vi "XVA-DSE1-dist.vi"(8 "err in":errorcluster, 10 "X-VA (e)":T2, 11 "p_LN":T1) -> (0 "err out":errorcluster, 2 "X-VA (s)":T2, 3 "p_LN (s)":T1)   [LabVIEW 2010, in "lv_04.lvlib"]
uses:
  lv_04.lvlib
  lv_02/p_5E1_LN.ctl
  commandes/cX.ctl
  commandes/cSTA_varid.ctl
  commandes/c_TDMS_ch_variable.ctl
  commandes/c_TDMS_ch_donnees.ctl
  commandes/c0-var-n.ctl
  commandes/cSTA_num_do_cr.ctl
  commandes/c02-do-num.ctl
  commandes/c04-stat-num.ctl
  commandes/cSTA_txt_do_cr.ctl
  commandes/c02-do-txt.ctl
  commandes/c04-stat-txt.ctl
  commandes/cSTA_dist.ctl
  commandes/c03-dist-S.ctl
  commandes/c0-dist-xy.ctl
  commandes/c03-dist-T.ctl
  commandes/c03-dist-SPC.ctl
  lv_02/1-x-dist.vi
  lv_02/lv_02.lvlib
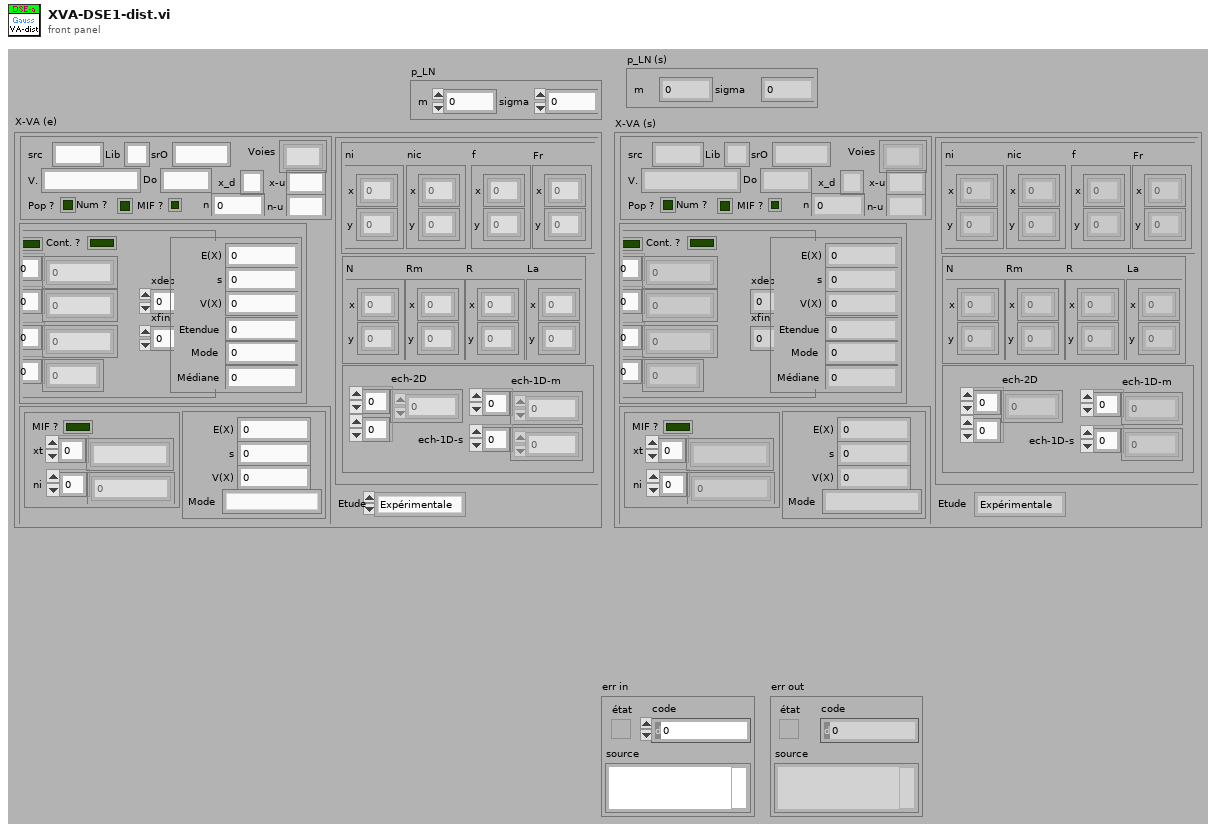
[diagram p1: front panel]
types:
  T1 = typedef "lv_02.lvlib/p_5E1_LN.ctl" = cluster{"m":dbl, "sigma":dbl}
  T2 = typedef "lv_04.lvlib/cX.ctl" = cluster{"src":T3, "num":T7, "txt":T10, "dist":T13, "Etude":enum16{"Expérimentale", "Modèle"}}
  T3 = typedef "lv_04.lvlib/cSTA_varid.ctl" = cluster{"src":string, "Lib":string, "srO":string, "V.":T4, "Voies":string[], "Do":T5, "n":T6, "Num ?":bool, "Pop ?":bool, "x_d":string, "x-u":string, "n-u":string, "MIF ?":bool}
  T4 = typedef "lv_04.lvlib/c_TDMS_ch_variable.ctl" = string
  T5 = typedef "lv_04.lvlib/c_TDMS_ch_donnees.ctl" = string
  T6 = typedef "lv_04.lvlib/c0-var-n.ctl" = i32
  T7 = typedef "lv_04.lvlib/cSTA_num_do_cr.ctl" = cluster{"do":T8, "sta":T9}
  T8 = typedef "lv_04.lvlib/c02-do-num.ctl" = cluster{"MIF ?":bool, "Cont. ?":bool, "xi":dbl[], "xic":dbl[], "ni":u32[], "dx":dbl[], "xdeb":dbl, "xfin":dbl}
  T9 = typedef "lv_04.lvlib/c04-stat-num.ctl" = cluster{"E(X)":dbl, "s":dbl, "V(X) ":dbl, "Etendue":dbl, "Mode":dbl, "Médiane":dbl}
  T10 = typedef "lv_04.lvlib/cSTA_txt_do_cr.ctl" = cluster{"do":T11, "sta":T12}
  T11 = typedef "lv_04.lvlib/c02-do-txt.ctl" = cluster{"xt":string[], "ni":dbl[], "MIF ?":bool}
  T12 = typedef "lv_04.lvlib/c04-stat-txt.ctl" = cluster{"E(X)":dbl, "s":dbl, "V(X) ":dbl, "Mode":string}
  T13 = typedef "lv_04.lvlib/cSTA_dist.ctl" = cluster{"S":T14, "T":T16, "spc":T17}
  T14 = typedef "lv_04.lvlib/c03-dist-S.ctl" = cluster{"nic":T15, "f":T15, "Fr":T15, "ni":T15}
  T15 = typedef "lv_04.lvlib/c0-dist-xy.ctl" = cluster{"x":dbl[], "y":dbl[]}
  T16 = typedef "lv_04.lvlib/c03-dist-T.ctl" = cluster{"N":T15, "Rm":T15, "R":T15, "La":T15}
  T17 = typedef "lv_04.lvlib/c03-dist-SPC.ctl" = cluster{"ech-2D":dbl[][], "ech-1D-m":dbl[], "ech-1D-s":dbl[]}
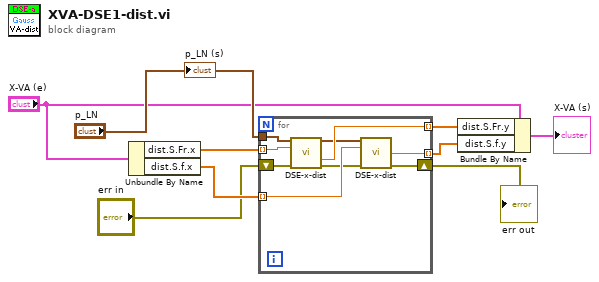
[diagram p0: block diagram]
diagram:
  n1 = Unbundle By Name("X-VA (e)") -> ("dist.S.Fr.x"=w9:dbl[], "dist.S.f.x"=w4:dbl[])
  n2 = for {
    tunnel: [w17] -> w6 mode=indexing
    tunnel: "p_LN" -> [w16]
    tunnel: w9 -> [w18] mode=indexing
    tunnel: w4 -> [w15] mode=indexing
    tunnel: [w14] -> w3 mode=indexing
    shift-right: [w10] -> w1
    shift-left: "err in" -> [w12]
    n3 = call-poly "DSE-x-dist.vi"("p_LN"=w16, "x"=w18, "error in"=w12) -> ("p_LN"=w13:T1, "F(x)"=w17:dbl, "error out"=w11:errorcluster)  [unwired: 8 in, 2 out]
    n4 = call-poly "DSE-x-dist.vi"("p_LN"=w13, "x"=w15, "error in"=w11) -> ("f(x)"=w14:dbl, "error out"=w10:errorcluster)  [unwired: 8 in, 3 out]
  }
  "err out" <- w1
  n5 = Bundle By Name(cluster="X-VA (e)", "dist.S.Fr.y"=w6, "dist.S.f.y"=w3) -> (→"X-VA (s)":T2)
  "p_LN (s)" <- "p_LN"
